vi "Step 6 - Postprocessing (NStageMRate).vi"() -> ()   [LabVIEW 2023]
doc: "Demonstrates how to use the DFD FXP NStage MRate Postprocessing VI to convert the filtered signal from a fixed-point integer representation to readable engineering unit values."
uses:
  <vilib>/addons/Digital Filter Design/_Objects.llb/DFD Multirate Filtering Mode.ctl
  <vilib>/addons/Digital Filter Design/_Objects.llb/DFD Multirate Filter Specification (Design).ctl
  <vilib>/addons/Digital Filter Design/_Objects.llb/DFD Coef Norm Type.ctl
  <vilib>/addons/Digital Filter Design/FXPMRateSim.llb/DFD FXP NStage MRate Simulation (DBL).vi
  <vilib>/addons/Digital Filter Design/FXPMRateSim.llb/DFD FXP NStage MRate Postprocessing (I32, 1Ch).vi
  <vilib>/addons/Digital Filter Design/NI_DigFilterLicensed.lvlib
  <vilib>/Analysis/NI_AALBase.lvlib
panel:
  out "Filtered Signals":dbl[][](graph)
  # "Select Help>>Show Context Help and move the cursor over the VI icon for more information."
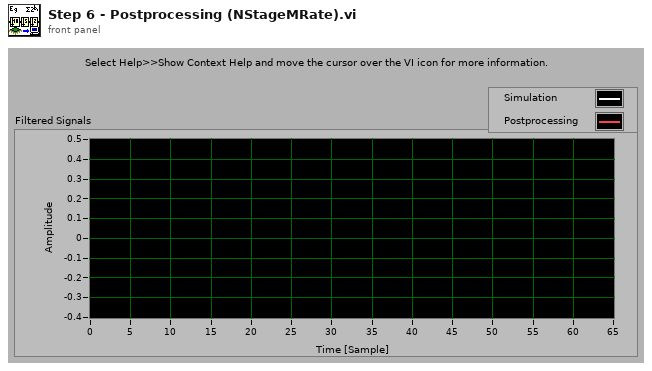
[diagram p1: front panel]
types:
  T1 = typedef "NI_DigFilterLicensed.lvlib/DFD Coef Norm Type.ctl" = enum16{"No Norm", "Time Domain 1-Norm", "Time Domain 2-Norm", "Time Domain Inf-Norm"}
  T2 = typedef "NI_DigFilterLicensed.lvlib/DFD Multirate Filter Specification (Design).ctl" = cluster{"fpass":dbl, "fstop":dbl}
  T3 = typedef "NI_DigFilterLicensed.lvlib/DFD Multirate Filtering Mode.ctl" = u16
  T4 = typedef "NI_DigFilterLicensed.lvlib/DFD Multirate Filter Obj.ctl" = cluster{"mMRate_Structure":enum16{"CIC", "FIR", "IIR", "Lattice"}, "mMRate_Mode":T5, "mMRate_Factor":i32, "mMRate_FIRParams":cluster{"mMRate_FIR_H":dbl[], "mMRate_FIR_IsNyquist?":bool, "mMRate_FIR_IsSymmetric?":bool}, "mMRate_CICParams":cluster{"mMRate_CIC_#Stage":i32, "mMRate_CIC_Lag":i32, "mMRate_CIC_Type":enum16{"Lowpass", "Highpass"}}, "mMRate_Order":i32, "mMRate_Version":string, "mMRate_Comments":string, "mMRate_RationalFactor":cluster{"mMRate_L":i32, "mMRate_M":i32}, "mMRate_Fs":dbl, "mMRate_Quantized?":bool, "mMRate_QFilterGain":dbl, "mMRate_CoefWl":i16, "mMRate_Scaling":cluster{"mMRate_ScaleByPowerOf2?":bool, "mMRate_ScaleType":T1}, "mMRate_InputWl":i16, "mMRate_OutputWl":i16, "mMRate_OutputMode":T6, "mMRate_MultMode":T7, "mMRate_BitPruning":bool, "mMRate_GainWl":i16, "mMRate_OutputFwl":i16, "mMRate_SumIwl":i16, "mMRate_InputIwl ":i16, "mMRate_SumWl":i16, "mMRate_CoefIwl":i16}
  T5 = typedef "NI_DigFilterLicensed.lvlib/DFD Multirate Mode.ctl" = i16
  T6 = typedef "NI_DigFilterLicensed.lvlib/DFD Round-off Mode.ctl" = enum16{"Nearest", "Truncation"}
  T7 = typedef "NI_DigFilterLicensed.lvlib/DFD FXP MRate Multiply Mode.ctl" = enum16{"Truncated", "Full"}
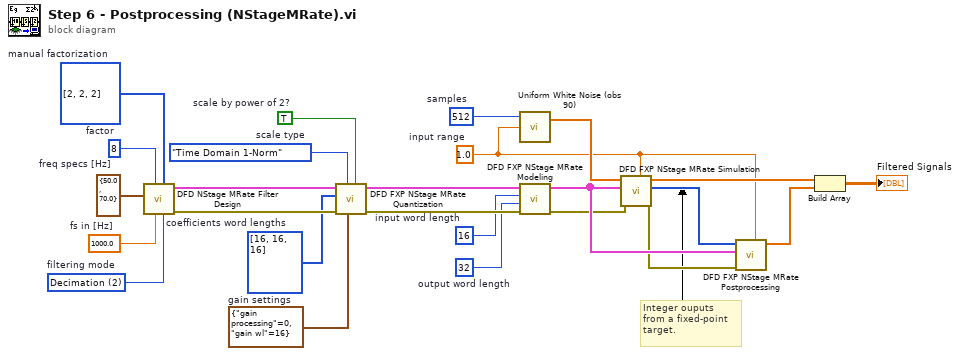
[diagram p0: block diagram]
diagram:
  w1 = i16 32  # output word length
  w2 = i16 16  # input word length
  w3 = i16[] [16, 16, 16]  # coefficients word lengths
  w6 = cluster{"gain processing":u16, "gain wl":i16} {"gain processing"=0, "gain wl"=16}  # gain settings
  w7 = 1.0  # input range
  w13 = 512  # samples
  w16 = TRUE  # scale by power of 2?
  w17 = DFD_Coef_Norm_Type."Time Domain 1-Norm"  # scale type
  w18 = 1000.0  # fs in [Hz]
  w19 = T2 {"fpass"=50.0, "fstop"=70.0}  # freq specs [Hz]
  w20 = i32[] [2, 2, 2]  # manual factorization
  w21 = 8  # factor
  w22 = T3 2 items=["No Rate Change", "Interpolation", "Decimation"]  # filtering mode
  # "Integer ouputs\nfrom a fixed-point\ntarget."
  n1 = call <vilib>:"DFD NStage MRate Filter Design.vi"("filtering mode"=w22, "manual factorization"=w20, "fs in [Hz]"=w18, "factor"=w21, "freq specs [Hz]"=w19) -> ("error out"=w11:errorcluster, "multirate filters out"=w12:T4[])  [unwired: 3 in, 2 out]
  n2 = call <vilib>:"DFD FXP NStage MRate Quantization.vi"("scale by power of 2? (F)"=w16, "gain settings"=w6, "scale type"=w17, "error in (no error)"=w11, "coefficients word lengths"=w3, "multirate filters in"=w12) -> ("error out"=w14:errorcluster, "multirate filters out"=w15:T4[])  [unwired: 4 out]
  n3 = call <vilib>:"Uniform White Noise (obs 90).vi"("amplitude"=w7, "samples"=w13) -> ("uniform white noise"=w10:dbl[])  [unwired: 1 in, 1 out]
  n4 = call <vilib>:"DFD FXP NStage MRate Modeling.vi"("error in (no error)"=w14, "output word length"=w1, "input word length"=w2, "multirate filters in"=w15) -> ("error out"=w5:errorcluster, "multirate filters out"=w9:T4[])  [unwired: 4 in, 2 out]
  n5 = call-poly <vilib>:"DFD FXP NStage MRate Simulation.vi"("input range"=w7, "error in (no error)"=w5, "multirate filters"=w9, "signal in"=w10) -> ("error out"=w4:errorcluster, "integer signal out"=w23:i32[], "DBL signal out"=w24:dbl[])  [unwired: 1 in, 4 out]
  n6 = call-poly <vilib>:"DFD FXP NStage MRate Postprocessing.vi"("input range"=w7, "error in (no error)"=w4, "multirate filters"=w9, "signal in"=w23) -> ("signal out"=w8:dbl[])  [unwired: 1 in, 6 out]
  n7 = Build Array(w24, w8) -> (→"Filtered Signals":dbl[][])
